vi "Mechanical Action Demo.vi"() -> ()   [LabVIEW 2010]
panel:
  out "Loop iteration":i32
  in  "Latch When Released":bool
  out "Boolean 9":bool
  out "Boolean 8":bool
  out "Boolean 7":bool
  in  "Latch Until Released":bool
  in  "Latch When Pressed":bool
  in  "stop":bool
  out "Boolean 6":bool
  out "Boolean 5":bool
  out "Boolean 4":bool
  in  "Switch Until Released":bool
  in  "Switch When Released":bool
  in  "Switch When Pressed":bool
  # "Switches to the new state as soon as\nthe button is pressed.  The \"Caps-Lock\"\non a keyboard is a good example of similar\nfunctionality."
  # "Switches to a new state as soon as the button is pressed, and retains the new value until the VI reads the value once.  Similar in functionality to a letter button (e.g., \"a\") on the keyboard."
  # "Same as above but the action only occurs\nafter the button is released."
  # "Same as above, but the action only occurs after the button is released."
  # "Switches to a new state as long as the\nbutton is held down and then reverts to\nits default value when you release it."
  # "Switches to a new state when you press it, and retains\nthe value until the VI reads it once or you release the\nbutton...depending on which occurs last."
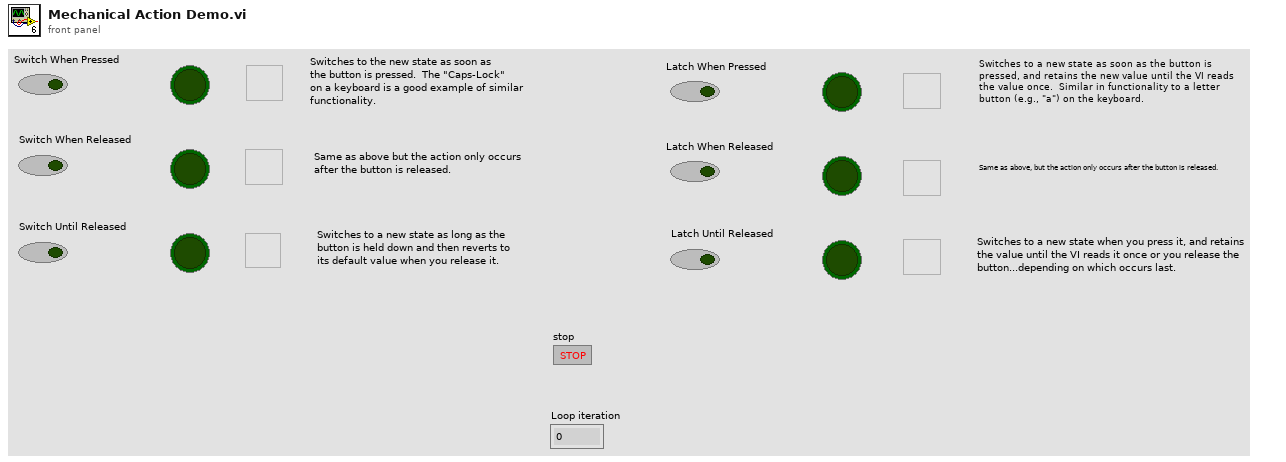
[diagram p1: front panel]
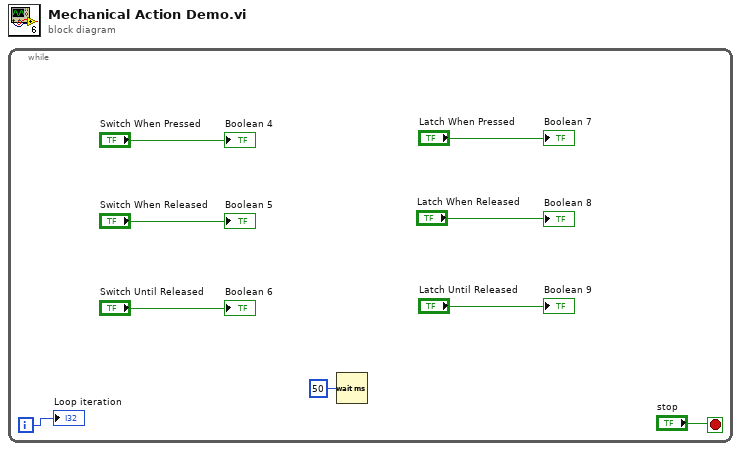
[diagram p0: block diagram]
diagram:
  n1 = while {
    i -> [w1]
    stop <- "stop" stop-if-true
    n2 = Wait (ms)(milliseconds to wait=u32 50) -> ()  [unwired: 1 out]
    "Boolean 4" <- "Switch When Pressed"
    "Boolean 5" <- "Switch When Released"
    "Boolean 6" <- "Switch Until Released"
    "Boolean 7" <- "Latch When Pressed"
    "Boolean 8" <- "Latch When Released"
    "Boolean 9" <- "Latch Until Released"
    "Loop iteration" <- w1
  }
